vi "Connection Listener Repository.vi"(8 "error in (no error)":errorcluster, 10 "Action(ReadRepository)":T1(ring), 11 "Websocket In":refnum<class "Websocket.lvclass">) -> (0 "error out":errorcluster, 1 "ProcessAlreadyStarted":bool, 2 "ToProcessQueue":refnum<queue>, 3 "Websocket Out":refnum<class "Websocket.lvclass">, 4 "ProcessSyncQueue":refnum<queue>, 5 "FromProcessQueue":refnum<queue>, 6 "ProcessViRef":refnum<vi>)   [LabVIEW 2017, in "Front Panel Publisher.lvlib" / "Websocket.lvclass"]
uses:
  Websocket.lvclass
  Connection Listener.ctl
panel:
  # "Use this indicator for sending messages to the Process VI"
  # "These indicators are used by the process VIs"
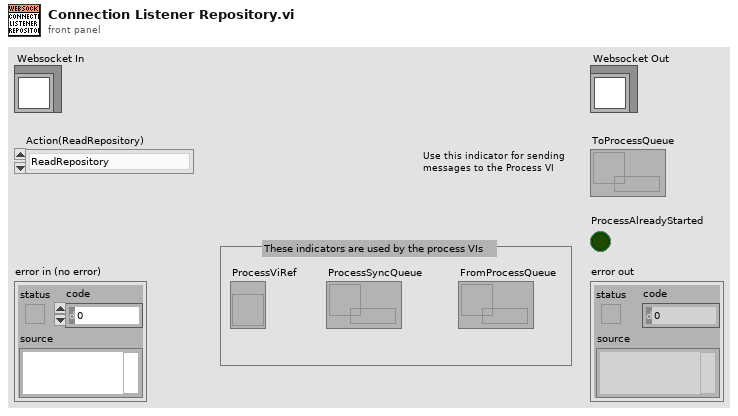
[diagram p1: front panel]
types:
  T1 = enum16{"ReadRepository", "CreateNew", "CreateOrLookUpExisting", "ReadRepositoryAndDestroy"}
  T2 = typedef "Front Panel Publisher.lvlib/Websocket.lvclass/Connection Listener.ctl" = cluster{"ToProcessQueue":refnum<queue>, "FromProcessQueue":refnum<queue>, "ProcessSyncQueue":refnum<queue>, "ProcessViRef":refnum<vi>}
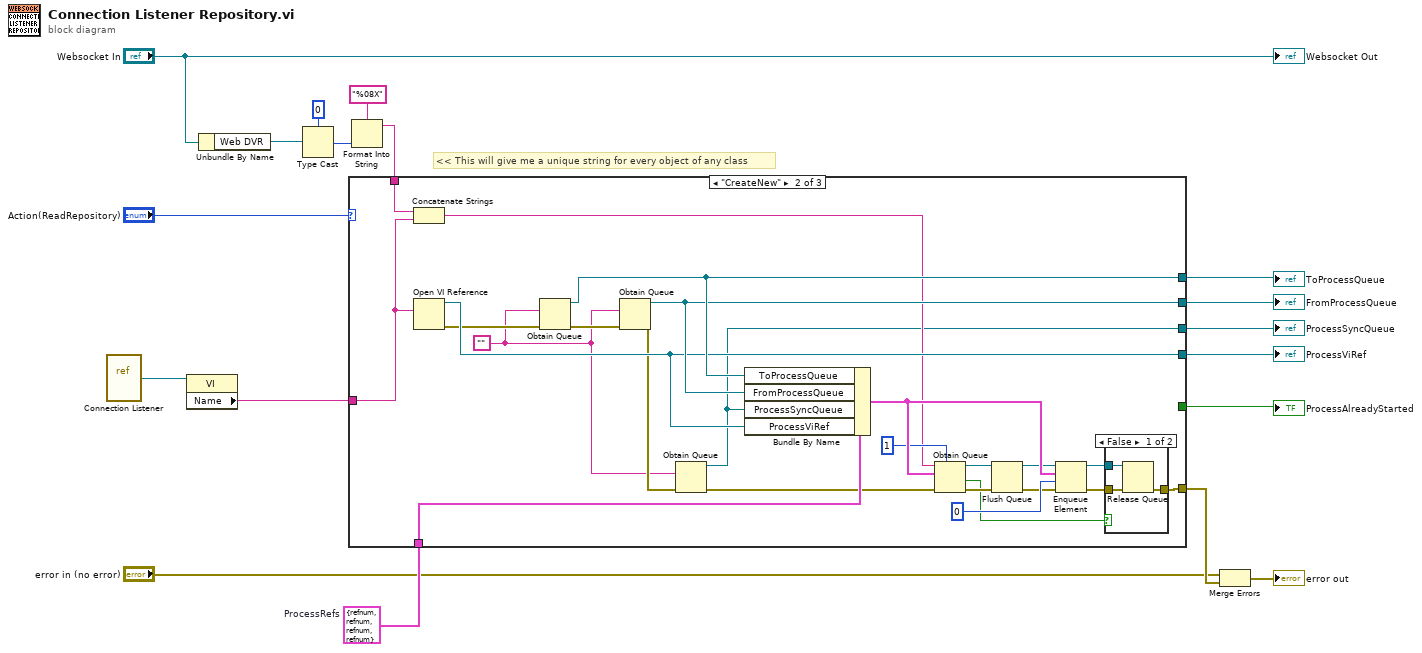
[diagram p0: block diagram]
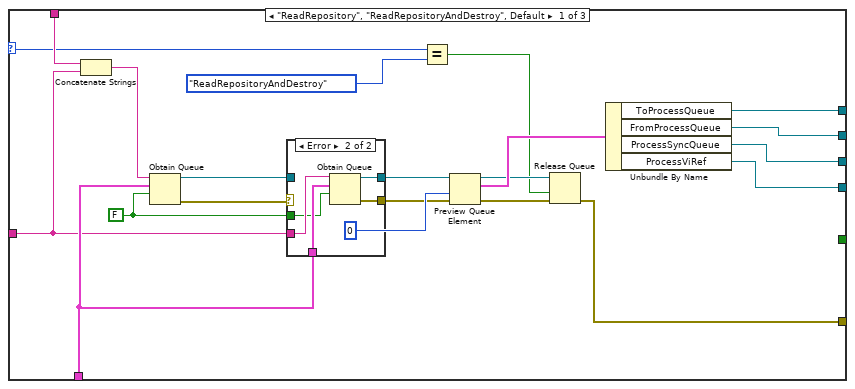
[diagram p2: hidden frame]
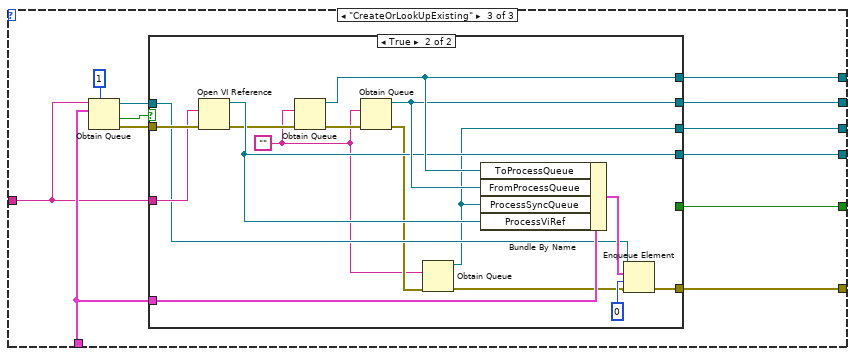
[diagram p5: hidden frame]
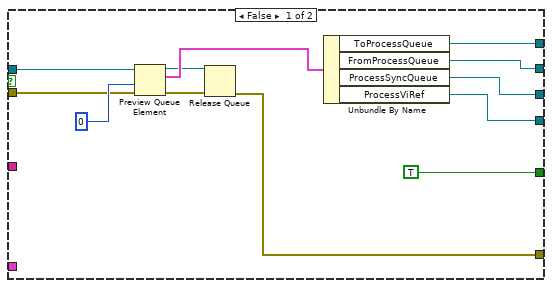
[diagram p6: hidden frame]
diagram:
  w13 = T2 {"ToProcessQueue"=refnum, "FromProcessQueue"=refnum, "ProcessSyncQueue"=refnum, "ProcessViRef"=refnum}  # ProcessRefs
  # "<< This will give me a unique string for every object of any class"
  n1 = vi-ref "Connection Listener.vi"() -> (w1:refnum<vi>)
  n2 = property class="VI"(reference=w1) -> ("Name"=w10:string)  [unwired: 1 in, 2 out]
  n3 = Unbundle By Name("Websocket In") -> ("Web DVR"=w2:refnum<data-value>)
  n4 = Type Cast(type=u32 0, x=w2) -> (*(type *) &x=w7:u32)
  n5 = Format Into String(format string="%08X", w7) -> (resulting string=w4:string)  [unwired: 2 in, 1 out]
  n6 = case shown="\"CreateNew\"" "Action(ReadRepository)" {
    selector: "Action(ReadRepository)" -> [w20 _ _]
    tunnel: [w34 w55 w84] -> w17
    tunnel: [w36 w70 w86] -> w15
    tunnel: [w35 w69 w85] -> w16
    tunnel: [w37 w68 w83] -> w14
    tunnel: w13 -> [w29 w61 w79]
    tunnel: w4 -> [w27 w60 _]
    tunnel: [w22 w48 w82] -> w11
    tunnel: w10 -> [w26 w58 w75]
    tunnel: [_ _ w77] -> w9
    frame "ReadRepository", "ReadRepositoryAndDestroy", Default {
      w28 = FALSE ("create if not found? (T)")
      n7 = Concatenate Strings(w27, w26) -> (w25:string)
      n8 = Obtain Queue(name (unnamed)=w25, element data type=w29, create if not found? (T)=w28) -> (queue out=w31:refnum<queue>, error out=w33:errorcluster)  [unwired: 2 in, 1 out]
      n9 = case shown="Error" w33 {
        selector: w33 -> [w41 _]
        tunnel: [w41 w43] -> w32
        tunnel: w31 -> [w40 _]
        tunnel: [w40 w44] -> w30
        tunnel: w29 -> [_ w46]
        tunnel: w26 -> [_ w45]
        tunnel: w28 -> [_ w42]
        frame No Error {
        }
        frame Error {
          n10 = Obtain Queue(name (unnamed)=w45, element data type=w46, create if not found? (T)=w42) -> (queue out=w44:refnum<queue>, error out=w43:errorcluster)  [unwired: 2 in, 1 out]
        }
      }
      n11 = Equal?(x=w20, y=T1."ReadRepositoryAndDestroy") -> (x = y?=w19:bool)
      n12 = Preview Queue Element(queue=w30, timeout in ms (-1)=0, error in (no error)=w32) -> (queue out=w24:refnum<queue>, element=w38:T2, error out=w23:errorcluster)  [unwired: 1 out]
      n13 = Release Queue(queue=w24, force destroy? (F)=w19, error in (no error)=w23) -> (error out=w22:errorcluster)  [unwired: 2 out]
      n14 = Unbundle By Name(w38) -> ("ToProcessQueue"=w36:refnum<queue>, "FromProcessQueue"=w35:refnum<queue>, "ProcessSyncQueue"=w34:refnum<queue>, "ProcessViRef"=w37:refnum<vi>)
    }
    frame "CreateNew" {
      w54 = ""
      n15 = Concatenate Strings(w60, w58) -> (w59:string)
      n16 = Open VI Reference(vi path=w58) -> (vi reference=w68:refnum<vi>, error out=w66:errorcluster)  [unwired: 5 in]
      n17 = Obtain Queue(element data type=w54, error in (no error)=w66) -> (queue out=w70:refnum<queue>, error out=w67:errorcluster)  [unwired: 3 in, 1 out]
      n18 = Obtain Queue(element data type=w54, error in (no error)=w67) -> (queue out=w69:refnum<queue>, error out=w57:errorcluster)  [unwired: 3 in, 1 out]
      n19 = Obtain Queue(element data type=w54, error in (no error)=w57) -> (queue out=w55:refnum<queue>, error out=w56:errorcluster)  [unwired: 3 in, 1 out]
      n20 = Bundle By Name(cluster=w61, "ToProcessQueue"=w70, "FromProcessQueue"=w69, "ProcessSyncQueue"=w55, "ProcessViRef"=w68) -> (w64:T2)
      n21 = Obtain Queue(max queue size (-1, unlimited)=1, name (unnamed)=w59, element data type=w64, error in (no error)=w56) -> (queue out=w65:refnum<queue>, created new?=w47:bool, error out=w52:errorcluster)  [unwired: 1 in]
      n22 = Flush Queue(queue=w65, error in (no error)=w52) -> (queue out=w53:refnum<queue>, error out=w51:errorcluster)  [unwired: 1 out]
      n23 = Enqueue Element(queue=w53, element=w64, timeout in ms (-1)=0, error in (no error)=w51) -> (queue out=w50:refnum<queue>, error out=w49:errorcluster)  [unwired: 1 out]
      n24 = case shown="False" w47 {
        tunnel: w49 -> [w73 w74]
        tunnel: w50 -> [w72 _]
        tunnel: [w71 w74] -> w48
        frame False {
          n25 = Release Queue(queue=w72, error in (no error)=w73) -> (error out=w71:errorcluster)  [unwired: 1 in, 2 out]
        }
        frame True {
        }
      }
    }
    frame "CreateOrLookUpExisting" {
      n26 = Obtain Queue(max queue size (-1, unlimited)=1, name (unnamed)=w75, element data type=w79) -> (queue out=w80:refnum<queue>, created new?=w81:bool, error out=w78:errorcluster)  [unwired: 2 in]
      n27 = case shown="True" w81 {
        tunnel: [w98 w114] -> w86
        tunnel: [w97 w113] -> w85
        tunnel: [w96 w99] -> w84
        tunnel: [w95 w112] -> w83
        tunnel: [w87 w111] -> w82
        tunnel: w79 -> [_ w110]
        tunnel: w78 -> [w92 w105]
        tunnel: w75 -> [_ w104]
        tunnel: w80 -> [w93 w103]
        tunnel: [TRUE _] -> w77
        frame False {
          n28 = Preview Queue Element(queue=w93, timeout in ms (-1)=0, error in (no error)=w92) -> (queue out=w89:refnum<queue>, element=w91:T2, error out=w88:errorcluster)  [unwired: 1 out]
          n29 = Release Queue(queue=w89, error in (no error)=w88) -> (error out=w87:errorcluster)  [unwired: 1 in, 2 out]
          n30 = Unbundle By Name(w91) -> ("ToProcessQueue"=w98:refnum<queue>, "FromProcessQueue"=w97:refnum<queue>, "ProcessSyncQueue"=w96:refnum<queue>, "ProcessViRef"=w95:refnum<vi>)
        }
        frame True {
          w100 = ""
          n31 = Open VI Reference(vi path=w104, error in (no error)=w105) -> (vi reference=w112:refnum<vi>, error out=w108:errorcluster)  [unwired: 4 in]
          n32 = Obtain Queue(element data type=w100, error in (no error)=w108) -> (queue out=w114:refnum<queue>, error out=w109:errorcluster)  [unwired: 3 in, 1 out]
          n33 = Obtain Queue(element data type=w100, error in (no error)=w109) -> (queue out=w113:refnum<queue>, error out=w102:errorcluster)  [unwired: 3 in, 1 out]
          n34 = Obtain Queue(element data type=w100, error in (no error)=w102) -> (queue out=w99:refnum<queue>, error out=w101:errorcluster)  [unwired: 3 in, 1 out]
          n35 = Bundle By Name(cluster=w110, "ToProcessQueue"=w114, "FromProcessQueue"=w113, "ProcessSyncQueue"=w99, "ProcessViRef"=w112) -> (w107:T2)
          n36 = Enqueue Element(queue=w103, element=w107, timeout in ms (-1)=0, error in (no error)=w101) -> (error out=w111:errorcluster)  [unwired: 2 out]
        }
      }
    }
  }
  "ProcessSyncQueue" <- w17
  "ToProcessQueue" <- w15
  "FromProcessQueue" <- w16
  "ProcessViRef" <- w14
  "ProcessAlreadyStarted" <- w9
  n37 = Merge Errors("error in (no error)", w11) -> (→"error out":errorcluster)
  "Websocket Out" <- "Websocket In"
